vi "CCT calculator per AMS.vi"(8 "CT_offset":dbl=1391.0 format="%#_13g", 9 "R'":dbl, 10 "B'":dbl, 11 "CT_coeff":dbl=3810.0 format="%#_13g") -> (2 "Color Temperature":dbl)   [LabVIEW 2014, in "AMS TS3472 Light Sensor.lvlib" / "AMS TCS3472.lvclass"]
uses:
  AMS TCS3472.lvclass
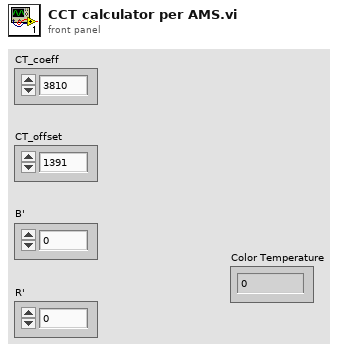
[diagram p1: front panel]
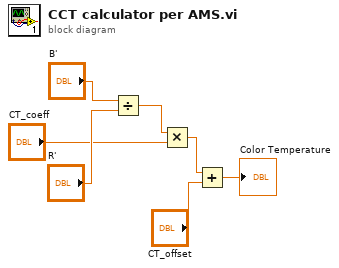
[diagram p0: block diagram]
diagram:
  n1 = Divide(x="B'", y="R'") -> (x/y=w5:dbl)
  n2 = Multiply(x=w5, y="CT_coeff") -> (x*y=w4:dbl)
  n3 = Add(x=w4, y="CT_offset") -> (x+y=→"Color Temperature":dbl)
